vi "Decimate Data For 2D Intensity Chart.vi"(9 "Plot Area":T1, 11 "2D Display in":u16[][](array[numeric])) -> (3 "Decimated Display":u16[][](array[numeric]))   [LabVIEW 2026, in "MicroPulse_Driver.lvlib"]
uses:
  MicroPulse_Driver.lvlib
  <vilib>/Utility/miscctls.llb/LVBoundsTypeDef.ctl
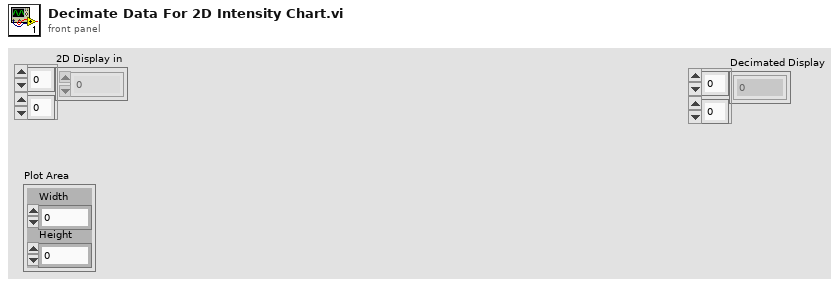
[diagram p1: front panel]
types:
  T1 = typedef "LVBoundsTypeDef.ctl" = cluster{"Width":u32, "Height":u32}
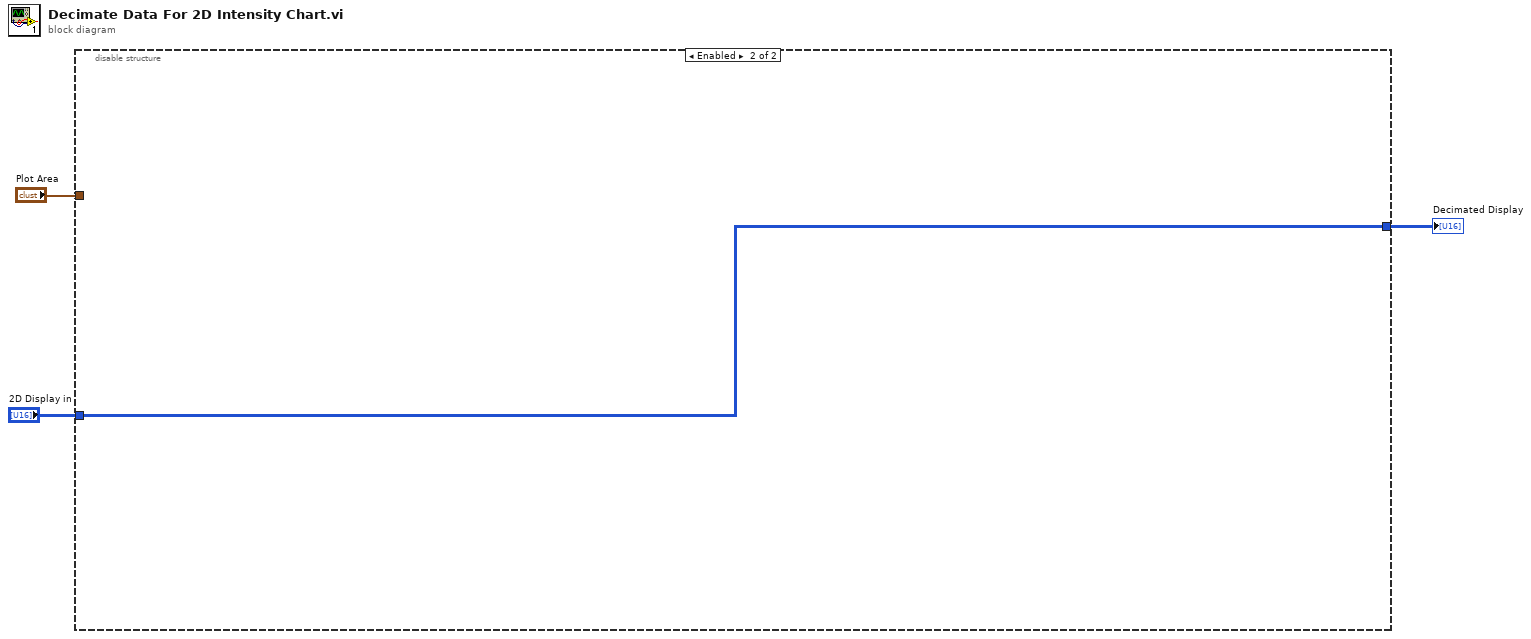
[diagram p0: block diagram]
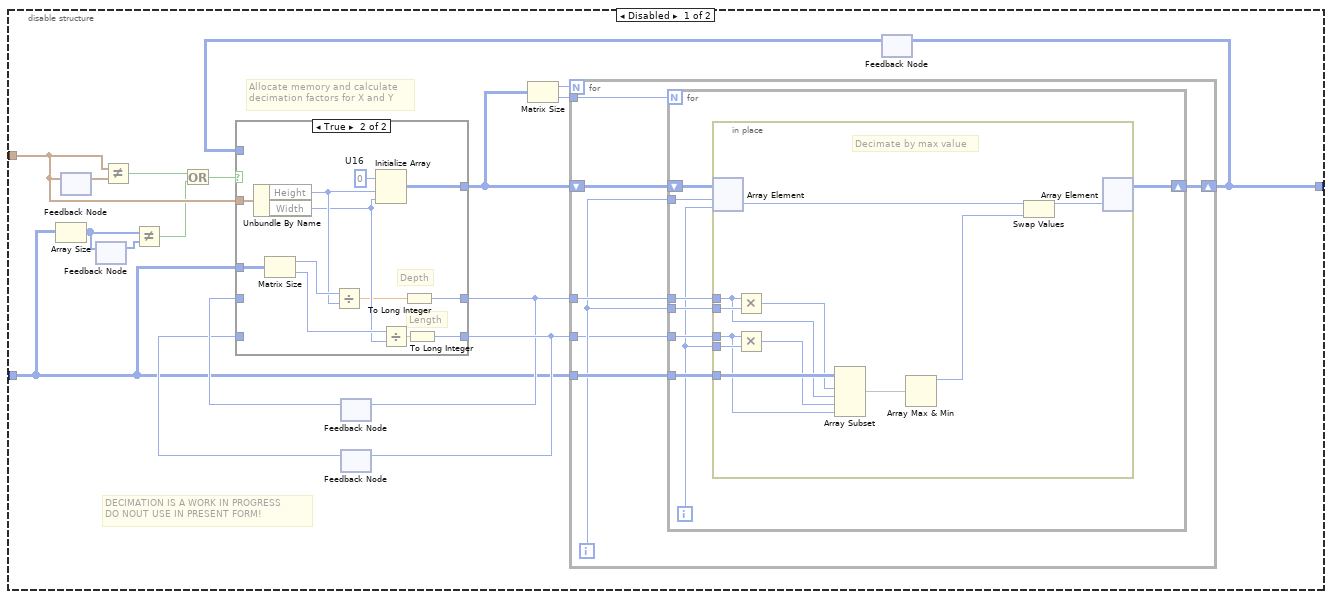
[diagram p2: hidden frame]
diagram:
  n1 = disable-structure shown="Enabled" {
    disable-tunnel: "Plot Area" -> [w18 _]
    disable-tunnel: [w17 w62] -> w2
    disable-tunnel: "2D Display in" -> [w8 w62]
    frame Disabled {
      # "DECIMATION IS A WORK IN PROGRESS\nDO NOUT USE IN PRESENT FORM!"
      # "Allocate memory and calculate\ndecimation factors for X and Y"
      n2 = Array Size(array=w8) -> (size(s)=w7:i32[])
      n3 = feedback #1() -> (w20:T1)  [unwired: 1 in]
      n4 = feedback-in #1(w18) -> ()
      n5 = feedback #2() -> (w6:i32[])  [unwired: 1 in]
      n6 = feedback-in #2(w7) -> ()
      n7 = Not Equal?(x=w18, y=w20) -> (x != y?=w19:bool)
      n8 = Not Equal?(x=w7, y=w6) -> (x != y?=w4:bool)
      n9 = Or(x=w19, y=w4) -> (x .or. y?=w5:bool)
      n10 = feedback #3() -> (w15:i32)  [unwired: 1 in]
      n11 = feedback #4() -> (w13:i32)  [unwired: 1 in]
      n12 = feedback #5() -> (w16:u16[][])  [unwired: 1 in]
      n13 = case shown="True" w5 {
        tunnel: w18 -> [_ w35]
        tunnel: [w23 w33] -> w11
        tunnel: w16 -> [w23 _]
        tunnel: w8 -> [_ w32]
        tunnel: [w22 w25] -> w12
        tunnel: [w21 w24] -> w14
        tunnel: w15 -> [w22 _]
        tunnel: w13 -> [w21 _]
        frame False {
        }
        frame True {
          w34 = u16 0  # U16
          # "Length"
          # "Depth"
          n14 = Unbundle By Name(w35) -> ("Height"=w30:u32, "Width"=w28:u32)
          n15 = Matrix Size(0:w32) -> (1:w31:i32, 2:w29:i32)
          n16 = Divide(x=w31, y=w30) -> (x/y=w27:dbl)
          n17 = Initialize Array(w34, w30, w28) -> (w33:u16[][])
          n18 = Divide(x=w29, y=w28) -> (x/y=w26:dbl)
          n19 = To Long Integer(number=w27) -> (32bit integer=w25:i32)
          n20 = To Long Integer(number=w26) -> (32bit integer=w24:i32)
        }
      }
      n21 = feedback-in #3(w12) -> ()
      n22 = feedback-in #4(w14) -> ()
      n23 = Matrix Size(0:w11) -> (1:w10:i32, 2:w9:i32)
      n24 = for {
        N: w10 -> [_]
        shift-right: [w41] -> w17
        shift-left: w11 -> [w42]
        tunnel: w8 -> [w40]
        tunnel: w12 -> [w39]
        tunnel: w14 -> [w37]
        tunnel: w9 -> [w36]
        i -> [w38]
        n25 = for {
          N: w36 -> [_]
          shift-right: [w49] -> w41
          shift-left: w42 -> [w50]
          tunnel: w38 -> [w48]
          tunnel: w40 -> [w47]
          tunnel: w39 -> [w46]
          tunnel: w38 -> [w45]
          tunnel: w37 -> [w44]
          i -> [w43]
          n26 = in-place {
            in-place-border: w47 -> [w61]
            in-place-border: w46 -> [w56]
            in-place-border: w45 -> [w59]
            in-place-border: w44 -> [w55]
            in-place-border: w43 -> [w58]
            # "Decimate by max value"
            n27 = in-place-array #6(w50, w48, w43) -> (w53:u16)
            n28 = Multiply(x=w56, y=w59) -> (x*y=w60:i32)
            n29 = Multiply(x=w55, y=w58) -> (x*y=w57:i32)
            n30 = Array Subset(array=w61, index (row)=w60, length (row)=w56, index (col)=w57, length (col)=w55) -> (w54:u16[][])
            n31 = Array Max & Min(array=w54) -> (max value=w52:u16)  [unwired: 3 out]
            n32 = Swap Values(12:w53, 14:w52) -> (1:w51:u16)  [unwired: 1 in, 1 out]
            n33 = in-place-array #6(w51) -> (w49:u16[][])  [unwired: 2 out]
          }
        }
      }
      n34 = feedback-in #5(w17) -> ()
    }
    frame Enabled {
    }
  }
  "Decimated Display" <- w2
